vi "双向脚本.vi"(0 "正向扫描电压(V)":dbl min=0.0 max=40.0 step=0.1, 1 "反向扫描电压(V)":dbl min=0.0 max=40.0 step=0.1, 2 "电压改变量":dbl, 3 "正向极限电流(mA)":dbl min=0.0 max=5.0 step=0.1, 4 "反向极限电流(mA)":dbl min=0.0 max=50.0 step=0.1) -> (7 "Script":string)   [LabVIEW 2019]
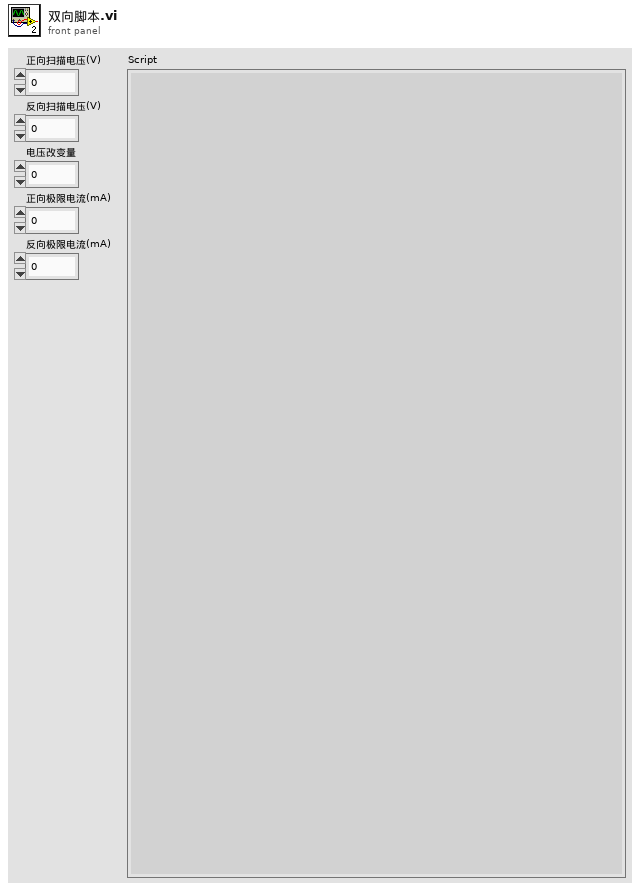
[diagram p1: front panel]
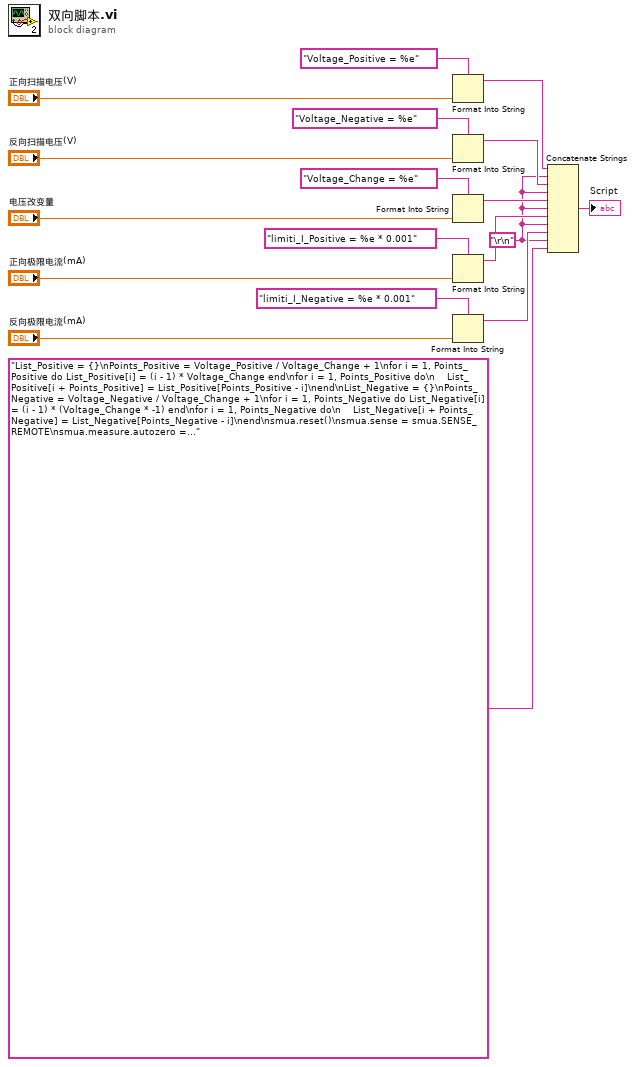
[diagram p0: block diagram]
diagram:
  w3 = "\r\n"
  n1 = Format Into String(format string="Voltage_Positive = %e" ("格式字符串"), "正向扫描电压(V)") -> (resulting string=w8:string)  [unwired: 2 in, 1 out]
  n2 = Format Into String(format string="Voltage_Negative = %e" ("格式字符串"), "反向扫描电压(V)") -> (resulting string=w7:string)  [unwired: 2 in, 1 out]
  n3 = Format Into String(format string="Voltage_Change = %e" ("格式字符串"), "电压改变量") -> (resulting string=w4:string)  [unwired: 2 in, 1 out]
  n4 = Format Into String(format string="limiti_I_Positive = %e * 0.001" ("格式字符串"), "正向极限电流(mA)") -> (resulting string=w6:string)  [unwired: 2 in, 1 out]
  n5 = Format Into String(format string="limiti_I_Negative = %e * 0.001" ("格式字符串"), "反向极限电流(mA)") -> (resulting string=w5:string)  [unwired: 2 in, 1 out]
  n6 = Concatenate Strings(w8, w3, w7, w3, w4, w3, w6, w3, w5, w3, "List_Positive = {}\nPoints_Positive = Voltage_Positive / Voltage_Change + 1\nfor i = 1, Points_Positive do List_Positive[i] = (i - 1) * Voltage_Change end\nfor i = 1, Points_Positive do\n    List_Positive[i + Points_Positive] = List_Positive[Points_Positive - i]\nend\nList_Negative = {}\nPoints_Negative = Voltage_Negative / Voltage_Change + 1\nfor i = 1, Points_Negative do List_Negative[i] = (i - 1) * (Voltage_Change * -1) end\nfor i = 1, Points_Negative do\n    List_Negative[i + Points_Negative] = List_Negative[Points_Negative - i]\nend\nsmua.reset()\nsmua.sense = smua.SENSE_REMOTE\nsmua.measure.autozero = smua.AUTOZERO_ONCE\nfunction init_Buffers()\n    local snvBuffers = {smua.nvbuffer1, smua.nvbuffer2}\n    for k, selBuffer in ipairs(snvBuffers) do\n        selBuffer.clear()\n        selBuffer.appendmode = 1\n        selBuffer.collecttimestamps = 1\n        selBuffer.collectsourcevalues = 1\n    end\nend\ninit_Buffers()\nsmua.source.output = smua.OUTPUT_ON\nsmua.source.limiti = limiti_I_Positive\nfor i, v in ipairs(List_Positive) do\n    smua.source.levelv = v\n    smua.measure.i(smua.nvbuffer1)\nend\nsmua.source.limiti = limiti_I_Negative\nfor i, v in ipairs(List_Negative) do\n    smua.source.levelv = v\n    smua.measure.i(smua.nvbuffer2)\nend\nsmua.source.leveli = 0\nsmua.source.levelv = 0\nsmua.source.output = smua.OUTPUT_OFF\nprint(\"{done}\")\nreset()") -> (→"Script":string)
